vi "Stop Core.vi"(10 "final error code":i32, 11 "Beep.lvclass in":refnum<class "Beep.lvclass">) -> (3 "Beep.lvclass out":refnum<class "Beep.lvclass">)   [LabVIEW 2016, in "CS++BeepActor.lvlib" / "Beep.lvclass"]
doc: "(<B>Filename</B>: Actor Framework.lvlib:Actor.lvclass:Stop Core.vi)\n\nDefines what the actor does before it stops. Use the <B>final error code</B> input to determine whether the actor shut down in response to an error.\n\nBy default, this method does nothing. A descendant class may override it to define behavior, such as shutting down any processes the actor initiated in its override of the Actor Core method."
uses:
  Beep.lvclass
  CSPP_Core/Actors/CS++BaseActor/CS++BaseActor.lvclass
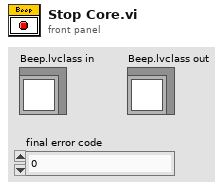
[diagram p1: front panel]
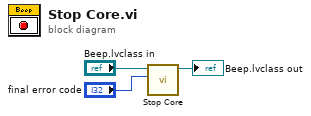
[diagram p0: block diagram]
diagram:
  n1 = call-parent "Stop Core.vi"("final error code"="final error code", "CS++BaseActor in"="Beep.lvclass in") -> ("CS++BaseActor out"=→"Beep.lvclass out":refnum<class "Beep.lvclass">)  [unwired: 9 in]
